vi "read_subtable_key_string.vi"(7 "subtables":string[](array[string]), 8 "error in (no error)":errorcluster, 9 "default (\"\")":string, 10 "subkeys":string[](array[string]), 11 "toml in":refnum<class "toml.lvclass">) -> (0 "error out":errorcluster, 1 "value":string="6.6.6", 2 "found?":bool, 3 "toml out":refnum<class "toml.lvclass">)   [LabVIEW 2020, in "toml.lvclass"]
uses:
  toml.lvclass
  toml.lvclass/toml.ctl
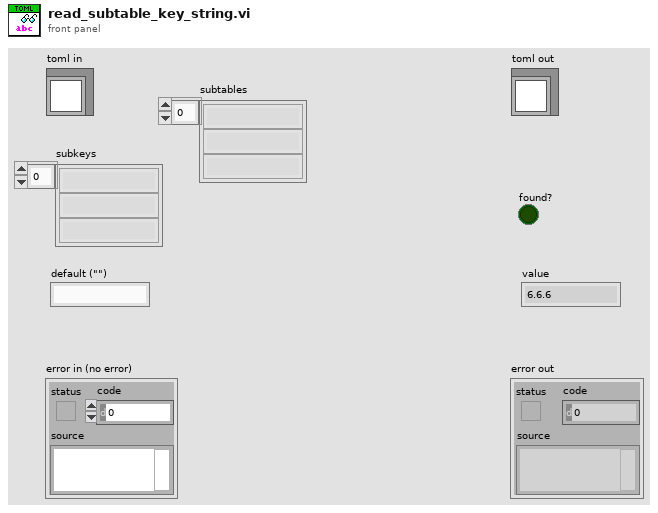
[diagram p1: front panel]
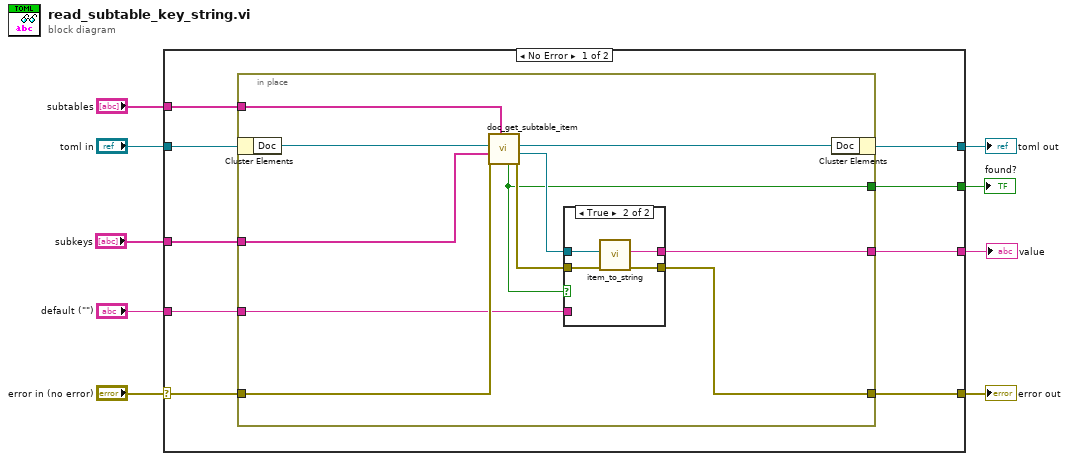
[diagram p0: block diagram]
diagram:
  n1 = case shown="No Error" "error in (no error)" {
    selector: "error in (no error)" -> [w12 w37]
    tunnel: [w13 w37] -> w8
    tunnel: [w17 w36] -> w6
    tunnel: "toml in" -> [w18 w36]
    tunnel: "subtables" -> [w16 _]
    tunnel: "subkeys" -> [w15 _]
    tunnel: "default (\"\")" -> [w14 _]
    tunnel: [w11 _] -> w2
    tunnel: [w10 _] -> w1
    frame No Error {
      n2 = in-place {
        in-place-border: w16 -> [w25]
        in-place-border: w15 -> [w29]
        in-place-border: w14 -> [w20]
        in-place-border: [w26] -> w13
        in-place-border: w12 -> [w28]
        in-place-border: [w21] -> w11
        in-place-border: [w19] -> w10
        n3 = in-place-cluster #1(w18) -> ("Doc"=w24:refnum<class "Doc.lvclass">)
        n4 = call "doc_get_subtable_item.vi"("subtables"=w25, "error in (no error)"=w28, "subkeys"=w29, "Doc in"=w24) -> ("error out"=w27:errorcluster, "item (value)"=w22:refnum<class "Item.lvclass">, "Doc out"=w23:refnum<class "Doc.lvclass">, "found?"=w19:bool)  [unwired: 4 in]
        n5 = case shown="True" w19 {
          tunnel: w27 -> [w31 w35]
          tunnel: [w31 w34] -> w26
          tunnel: w22 -> [_ w33]
          tunnel: [w30 w32] -> w21
          tunnel: w20 -> [w30 _]
          frame False {
          }
          frame True {
            n6 = call "item_to_string.vi"("error in (no error)"=w35, "Item in"=w33) -> ("error out"=w34:errorcluster, "string_value"=w32:string)  [unwired: 8 in]
          }
        }
        n7 = in-place-cluster #1("Doc"=w23) -> (w17:refnum<class "toml.lvclass">)
      }
    }
    frame Error {
    }
  }
  "error out" <- w8
  "toml out" <- w6
  "value" <- w2
  "found?" <- w1
